vi "ReadAimingBeamSetting.vi"(8 "error in (no error)":errorcluster) -> (0 "error out":errorcluster, 3 "Aiming Beam Setting":T1={"Aiming Beam COM Port"="COM3", "Min Current"=0.0, "Max Current"=63.0, "Default Current"=20.0, "Frequency(Hz)"=15})   [LabVIEW 2019]
uses:
  AimingBeam.ctl
  <vilib>/Utility/file.llb/Read Delimited Spreadsheet (string).vi
  <vilib>/addons/_JKI.lib/Serialization/JSON/JKI JSON Serialization.lvlib
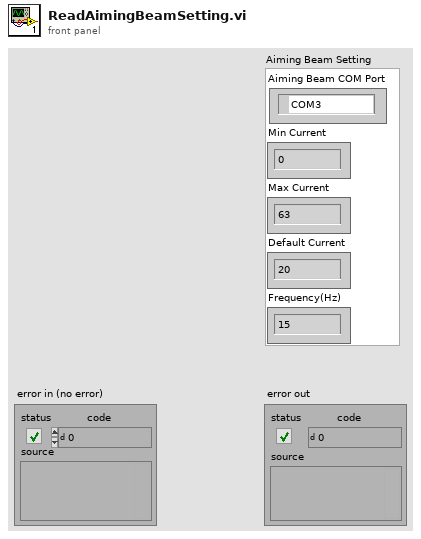
[diagram p1: front panel]
types:
  T1 = typedef "AimingBeam.ctl" = cluster{"Aiming Beam COM Port":refnum<visa-resource-name>, "Min Current":dbl, "Max Current":dbl, "Default Current":dbl, "Frequency(Hz)":u32}
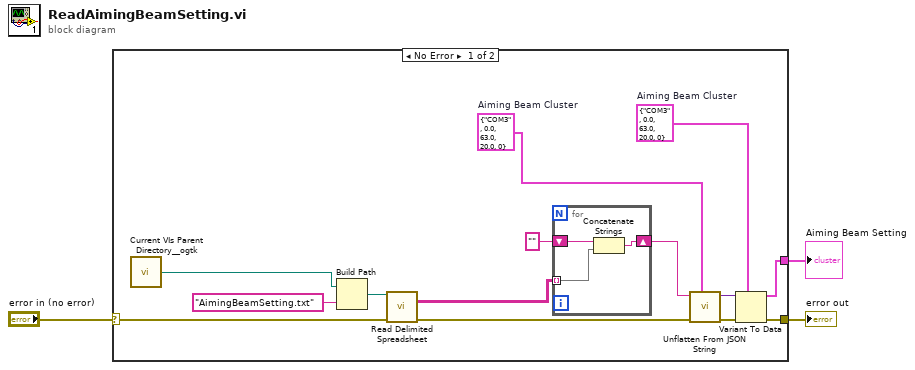
[diagram p0: block diagram]
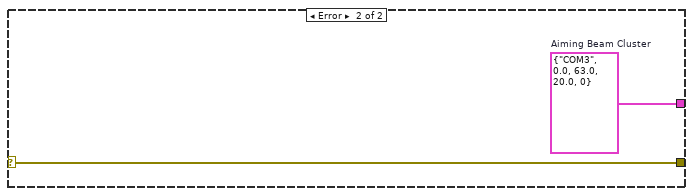
[diagram p2: hidden frame]
diagram:
  n1 = case shown="No Error" "error in (no error)" {
    selector: "error in (no error)" -> [w10 w22]
    tunnel: [w8 w22] -> w2
    tunnel: [w5 w21] -> w1
    frame No Error {
      w4 = T1 {"Aiming Beam COM Port"="COM3", "Min Current"=0.0, "Max Current"=63.0, "Default Current"=20.0, "Frequency(Hz)"=0}  # Aiming Beam Cluster
      w6 = T1 {"Aiming Beam COM Port"="COM3", "Min Current"=0.0, "Max Current"=63.0, "Default Current"=20.0, "Frequency(Hz)"=0}  # Aiming Beam Cluster
      n2 = call <userlib>:"Current VIs Parent Directory__ogtk.vi"() -> ("Parent Directory (+ Relative)"=w17:path)  [unwired: 5 in]
      n3 = Build Path(base path=w17, name or relative path="AimingBeamSetting.txt") -> (appended path=w15:path)
      n4 = call-poly <vilib>:"Read Delimited Spreadsheet.vi"("file path (dialog if empty)"=w15, "error in (no error)"=w10) -> ("all rows"=w13:string[][], "error out"=w11:errorcluster)  [unwired: 8 in, 4 out]
      n5 = for {
        tunnel: w13 -> [w20] mode=indexing
        shift-right: [w18] -> w12
        shift-left: "" -> [w19]
        n6 = Concatenate Strings(w19, w20) -> (w18:string)
      }
      n7 = call <vilib>:"Unflatten From JSON String.vi"("Type and Defaults"=w4, "error in (no error)"=w11, "JSON String"=w12) -> ("error out"=w9:errorcluster, "Variant"=w7:variant)  [unwired: 7 in]
      n8 = Variant To Data(error in=w9, type=w6, Variant=w7) -> (data=w5:T1, error out=w8:errorcluster)
    }
    frame Error {
      w21 = T1 {"Aiming Beam COM Port"="COM3", "Min Current"=0.0, "Max Current"=63.0, "Default Current"=20.0, "Frequency(Hz)"=0}  # Aiming Beam Cluster
    }
  }
  "error out" <- w2
  "Aiming Beam Setting" <- w1
